vi "SetCustomer.vi"(8 "Error In":errorcluster, 10 "Customer":refnum<class "Colleague.lvclass">, 11 "reference in":refnum<class "ManagerMediator.lvclass">) -> (0 "Error Out":errorcluster, 3 "reference in":refnum<class "ManagerMediator.lvclass">)   [LabVIEW 2020, in "ManagerMediator.lvclass"]
uses:
  ManagerMediator.lvclass
  Colleague_class/Colleague.lvclass
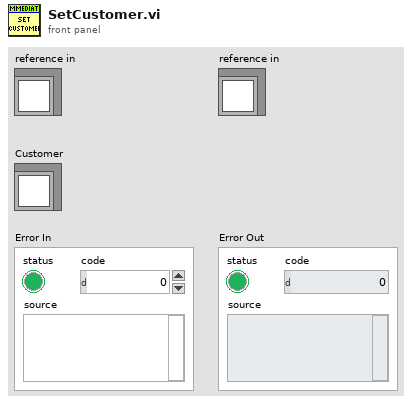
[diagram p1: front panel]
types:
  T1 = typedef "ManagerMediator.lvclass/ObjectAttributes.ctl" = cluster{"Customer":refnum<class "Colleague.lvclass">, "Programmer":refnum<class "Colleague.lvclass">, "Tester":refnum<class "Colleague.lvclass">}
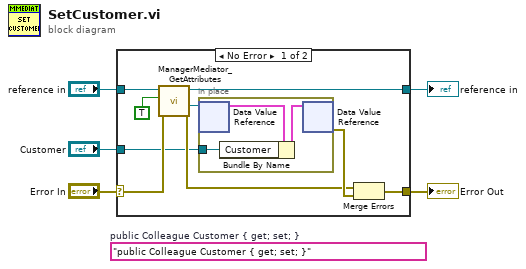
[diagram p0: block diagram]
diagram:
  (unwired) "public Colleague Customer { get; set; }"  # public Colleague Customer { get; set; }
  n1 = case shown="No Error" "Error In" {
    selector: "Error In" -> [w14 w19]
    tunnel: [w11 w19] -> w4
    tunnel: [w9 w18] -> w2
    tunnel: "reference in" -> [w10 w18]
    tunnel: "Customer" -> [w6 _]
    frame No Error {
      n2 = call "ManagerMediator_GetAttributes.vi"("error in (no error)"=w14, "OnlyGetDvrReference(False)"=TRUE, "reference in"=w10) -> ("error out"=w12:errorcluster, "DataRef"=w7:refnum<data-value>, "reference out"=w9:refnum<class "ManagerMediator.lvclass">)  [unwired: 5 in, 1 out]
      n3 = in-place {
        in-place-border: w6 -> [w17]
        n4 = in-place-dvr #1(w7) -> (w16:T1)  [unwired: 1 out]
        n5 = Bundle By Name(cluster=w16, "Customer"=w17) -> (w15:T1)
        n6 = in-place-dvr #1(w15) -> (w13:errorcluster)  [unwired: 1 out]
      }
      n7 = Merge Errors(w12, w13) -> (w11:errorcluster)
    }
    frame Error {
    }
  }
  "Error Out" <- w4
  "reference in" <- w2
